vi "Recipe_Editor.vi"() -> ()   [LabVIEW 2014]
uses:
  <vilib>/Utility/miscctls.llb/LVBoundsTypeDef.ctl
  <vilib>/Utility/file.llb/Read From Spreadsheet File (string).vi
panel:
  in  "Add Button":bool
  in  "Stop Button":bool
  in  "Open Button":bool
  in  "Recipe_Board":string[](tree)
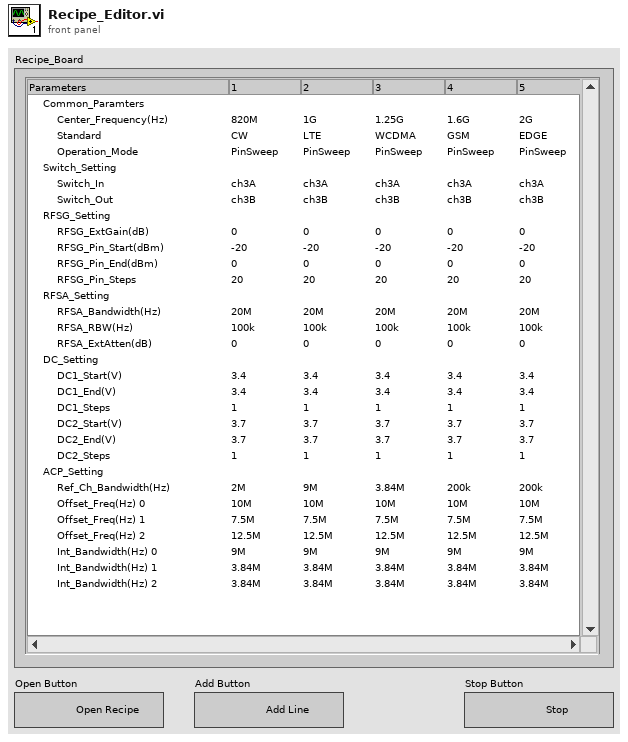
[diagram p1: front panel]
types:
  T1 = typedef "LVBoundsTypeDef.ctl" = cluster{"Width":u32, "Height":u32}
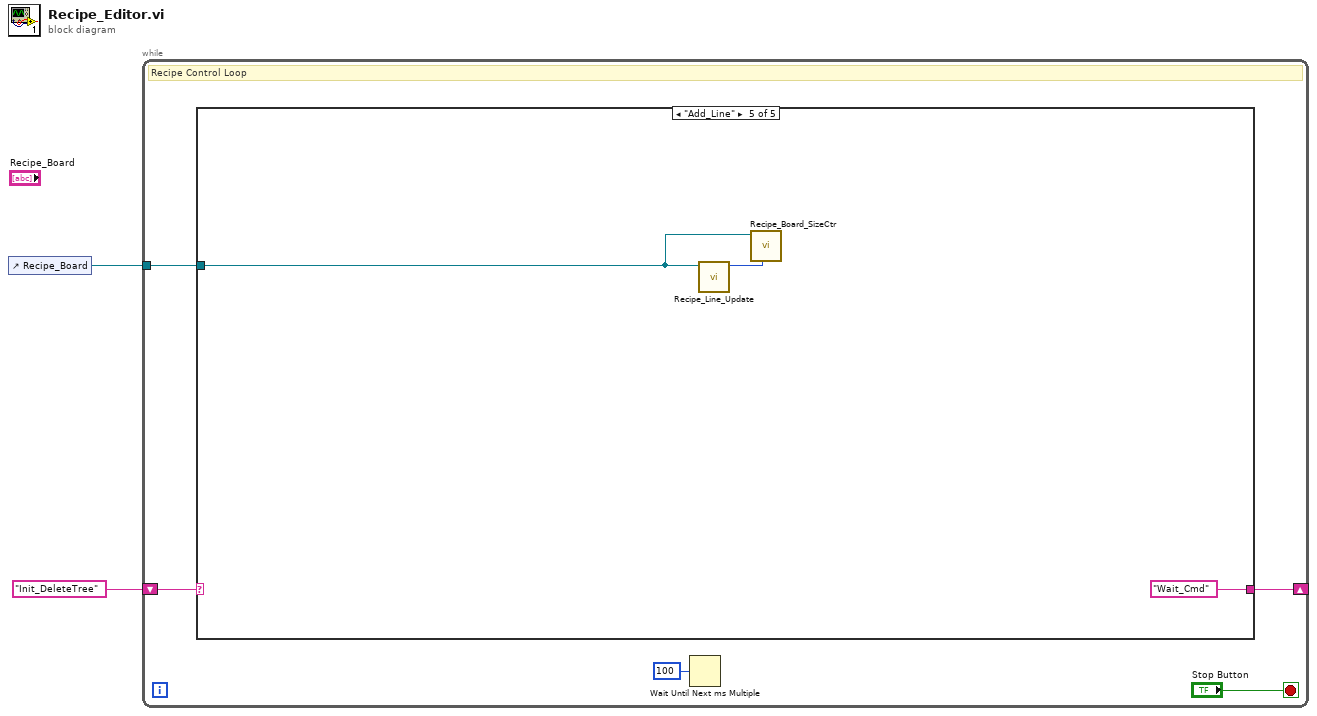
[diagram p0: block diagram]
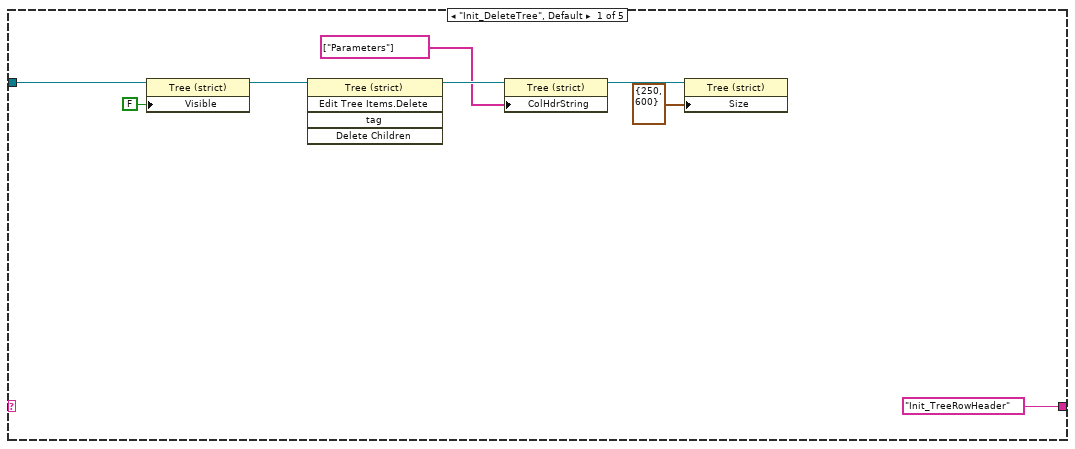
[diagram p2: hidden frame]
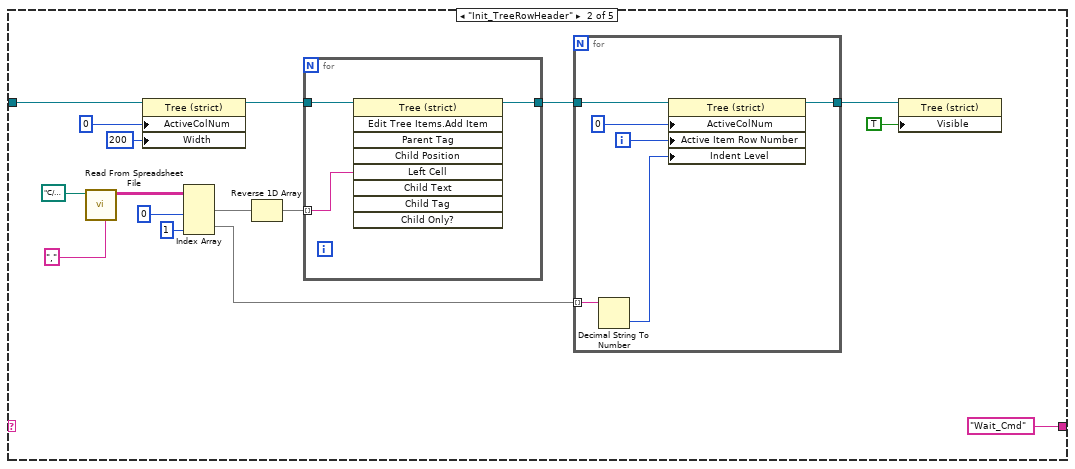
[diagram p3: hidden frame]
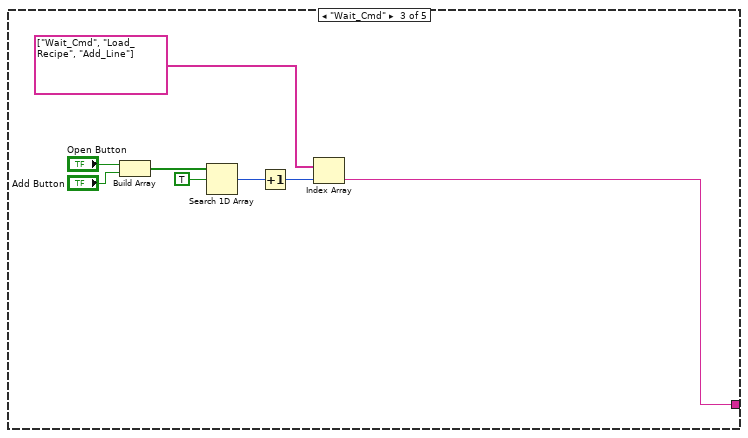
[diagram p4: hidden frame]
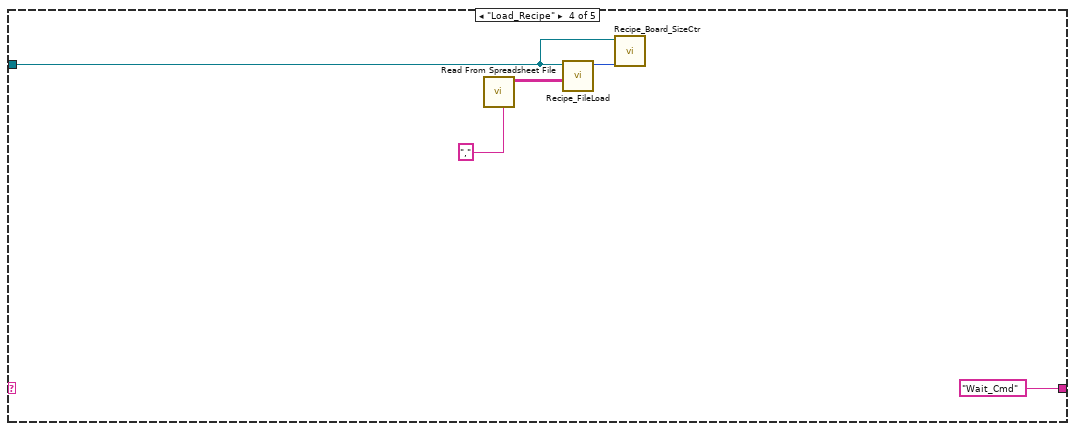
[diagram p5: hidden frame]
diagram:
  n1 = control-ref of="Recipe_Board"() -> (w1:refnum<vi>)
  n2 = while {
    shift-right: [w4] -> _
    shift-left: "Init_DeleteTree" -> [w6]
    tunnel: w1 -> [w5]
    stop <- "Stop Button" stop-if-true
    # "Recipe Control Loop"
    n3 = case shown="\"Add_Line\"" w6 {
      tunnel: w5 -> [w10 w17 _ w50 w55]
      tunnel: ["Init_TreeRowHeader" "Wait_Cmd" w41 "Wait_Cmd" "Wait_Cmd"] -> w4
      frame "Init_DeleteTree", Default {
        n4 = property class="Tree (strict)"(reference=w10, "Visible"=FALSE) -> (reference out=w8:refnum<vi>)  [unwired: 1 in, 1 out]
        n5 = invoke class="Tree (strict)" method="Edit Tree Items.Delete"(reference=w8) -> (reference out=w14:refnum<vi>)  [unwired: 4 in, 4 out]
        n6 = property class="Tree (strict)"(reference=w14, "ColHdrString"=string[] ["Parameters"]) -> (reference out=w12:refnum<vi>)  [unwired: 1 in, 1 out]
        n7 = property class="Tree (strict)"(reference=w12, "Size"=T1 {"Width"=250, "Height"=600}) -> ()  [unwired: 1 in, 2 out]
      }
      frame "Init_TreeRowHeader" {
        n8 = call-poly <vilib>:"Read From Spreadsheet File.vi"("delimiter (\\t)"="," ("delimiter (\\t)"), "file path (dialog if empty)"=path "C:/Gyuwon_Folder/SourceCodeFolder/1005_Gyu_RF_SourceProject_Msg/___SystemFiles/Recipe_Header.csv") -> ("all rows"=w28:string[][])  [unwired: 5 in, 4 out]
        n9 = property class="Tree (strict)"(reference=w17, "ActiveColNum"=0 ("Active Cell:Active Column Number"), "Width"=200 ("Active Cell:Cell Size:Width")) -> (reference out=w16:refnum<vi>)  [unwired: 1 in, 1 out]
        n10 = Index Array(array=w28, index (col) #1=0 ("disabled index (col)"), index (col) #2=1 ("index (col)")) -> (element #1=w26:string[], element #2=w24:string[])  [unwired: 2 in]
        n11 = Reverse 1D Array(array=w26) -> (reversed array=w29:string[])
        n12 = for {
          tunnel: w29 -> [w40] mode=indexing
          tunnel: [w39] -> w23
          tunnel: w16 -> [w38]
          n13 = invoke class="Tree (strict)" method="Edit Tree Items.Add Item"(reference=w38, "Left Cell"=w40) -> (reference out=w39:refnum<vi>)  [unwired: 7 in, 8 out]
        }
        n14 = for {
          tunnel: w23 -> [w37]
          tunnel: w24 -> [w34] mode=indexing
          tunnel: [w32] -> w20
          i -> [w35]
          n15 = Decimal String To Number(string=w34) -> (number=w33:i32)  [unwired: 2 in, 1 out]
          n16 = property class="Tree (strict)"(reference=w37, "ActiveColNum"=0 ("Active Cell:Active Column Number"), "Active Item Row Number"=w35, "Indent Level"=w33) -> (reference out=w32:refnum<vi>)  [unwired: 1 in, 1 out]
        }
        n17 = property class="Tree (strict)"(reference=w20, "Visible"=TRUE) -> ()  [unwired: 1 in, 2 out]
      }
      frame "Wait_Cmd" {
        n18 = Build Array("Open Button", "Add Button") -> (w46:bool[])
        n19 = Search 1D Array(1D array=w46, element=TRUE) -> (index of element=w44:i32)  [unwired: 1 in]
        n20 = Increment(x=w44) -> (x+1=w43:i32)
        n21 = Index Array(array=string[] ["Wait_Cmd", "Load_Recipe", "Add_Line"], index=w43) -> (element=w41:string)
      }
      frame "Load_Recipe" {
        n22 = call-poly <vilib>:"Read From Spreadsheet File.vi"("delimiter (\\t)"="," ("delimiter (\\t)")) -> ("all rows"=w51:string[][])  [unwired: 6 in, 4 out]
        n23 = call "Recipe_FileLoad.vi"("Recipe_Arr_From_File"=w51, "Recipe_Board_Ref"=w50) -> ("Recipe_Index"=w49:i32)  [unwired: 9 in]
        n24 = call "Recipe_Board_SizeCtr.vi"("Recipe_Index"=w49, "Recipe_Board_Ref"=w50) -> ()  [unwired: 10 in]
      }
      frame "Add_Line" {
        n25 = call "Recipe_Line_Update.vi"("Recipe_Board_Ref"=w55) -> ("Recipe_Index"=w54:i32)  [unwired: 10 in]
        n26 = call "Recipe_Board_SizeCtr.vi"("Recipe_Index"=w54, "Recipe_Board_Ref"=w55) -> ()  [unwired: 10 in]
      }
    }
    n27 = Wait Until Next ms Multiple(millisecond multiple=u32 100) -> ()  [unwired: 1 out]
  }
